vi "Get Active Structure If function.vi"(0 "Structure If Else in":refnum<class "Structure If Else.lvclass">, 11 "error in (no error)":errorcluster) -> (4 "Structure If Else out":refnum<class "Structure If Else.lvclass">, 6 "function list":T1, 15 "error out":errorcluster)   [LabVIEW 2016, in "Structure If Else.lvclass"]
uses:
  Structure If Else.lvclass
  E:/Repository/LabVIEW Script Language/source code/LSL components/functions/functionsbase/functionbase.lvclass
  function list.ctl
  functionsbase/functionbase.lvclass
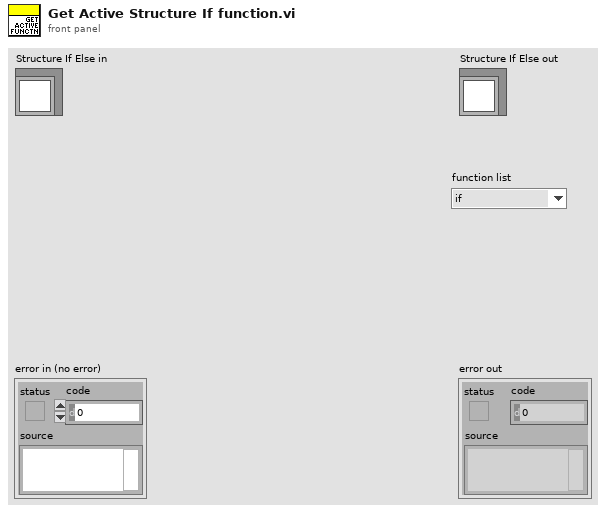
[diagram p1: front panel]
types:
  T1 = typedef "Structure If Else.lvclass/function list.ctl" = enum16{"if", "elif", "else"}
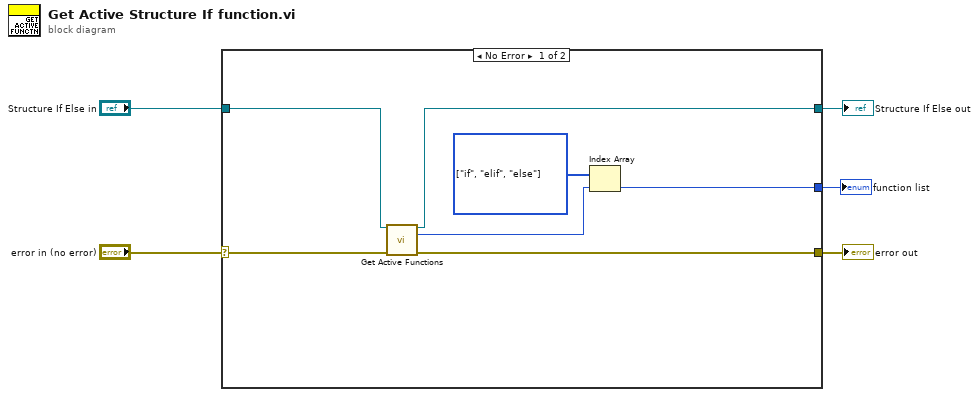
[diagram p0: block diagram]
diagram:
  n1 = case shown="No Error" "error in (no error)" {
    selector: "error in (no error)" -> [w12 w14]
    tunnel: [w11 w14] -> w4
    tunnel: [w9 w13] -> w2
    tunnel: "Structure If Else in" -> [w10 w13]
    tunnel: [w6 _] -> w1
    frame No Error {
      w7 = T1[] [enum."if", enum."elif", enum."else"] items=["if", "elif", "else"]
      n2 = call "Get Active Functions.vi"("functionbase in"=w10, "error in (no error)"=w12) -> ("functionbase out"=w9:refnum<class "Structure If Else.lvclass">, "Syntax Index"=w8:i32, "error out"=w11:errorcluster)  [unwired: 11 in]
      n3 = Index Array(array=w7, index=w8) -> (element=w6:T1)
    }
    frame Error {
    }
  }
  "error out" <- w4
  "Structure If Else out" <- w2
  "function list" <- w1
